vi "Refresh Limit Line.vi"(8 "error in (no error)":errorcluster, 10 "Item Names":string[][](array[string]), 11 "XY Graph":refnum<vi>) -> (0 "error out":errorcluster)   [LabVIEW 2020]
panel:
  out "XY Graph":cluster{dbl[], dbl[]}[](graph)
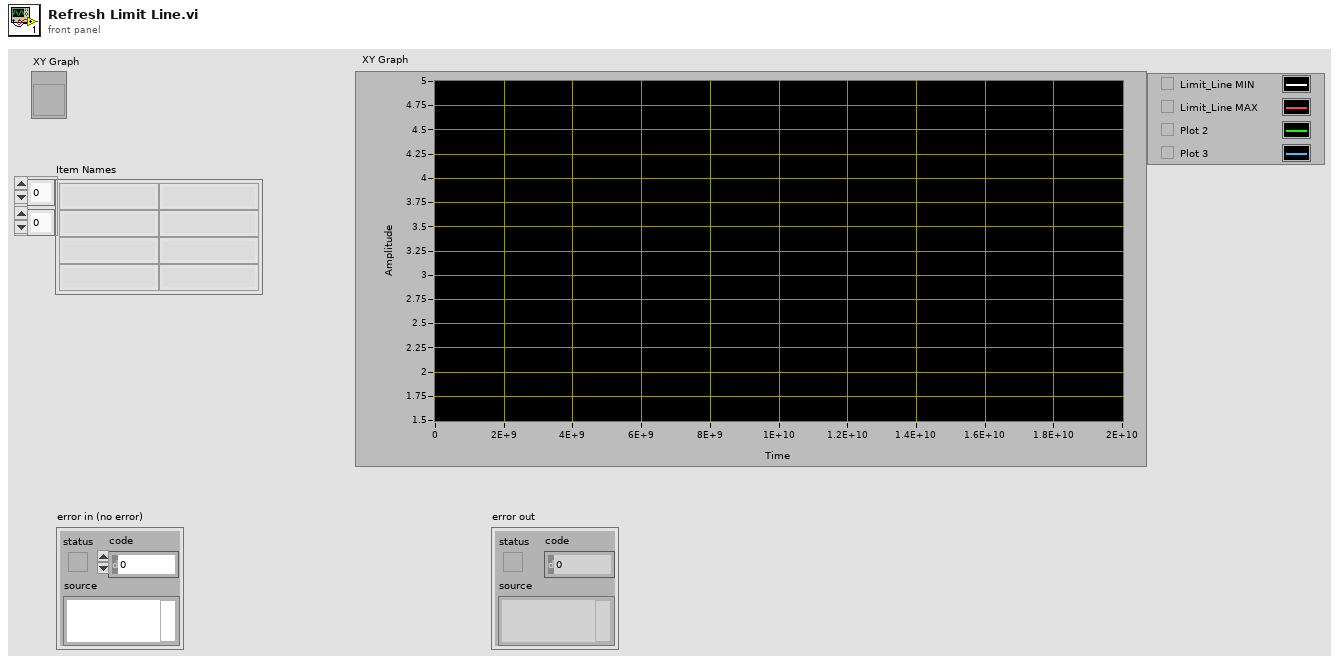
[diagram p1: front panel]
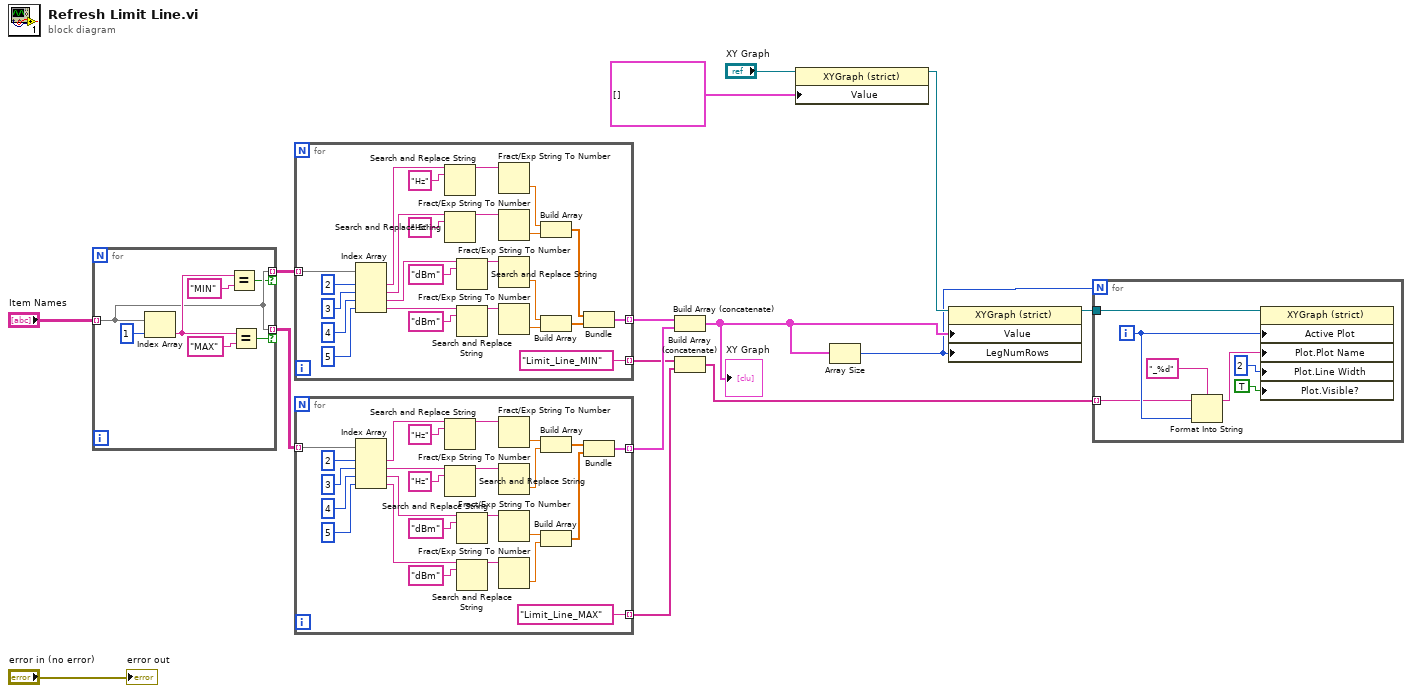
[diagram p0: block diagram]
diagram:
  n1 = for {
    tunnel: "Item Names" -> [w17] mode=indexing
    tunnel: [w17] -> w14 mode=indexing if=w20
    tunnel: [w17] -> w15 mode=indexing if=w16
    n2 = Index Array(array=w17, index=1) -> (element=w19:string)
    n3 = Equal?(x=w19, y="MIN") -> (x = y?=w16:bool)
    n4 = Equal?(x=w19, y="MAX") -> (x = y?=w20:bool)
  }
  n5 = for {
    tunnel: w15 -> [w47] mode=indexing
    tunnel: [w24] -> w6 mode=indexing
    tunnel: ["Limit_Line_MIN" ("format string")] -> w3 mode=indexing
    n6 = Index Array(array=w47, index #1=2 ("index"), index #2=3 ("index"), index #3=4 ("index"), index #4=5 ("index")) -> (element #1=w44:string, element #2=w39:string, element #3=w29:string, element #4=w28:string)
    n7 = Search and Replace String(input string=w44, search string="Hz") -> (result string=w42:string)  [unwired: 6 in, 3 out]
    n8 = Search and Replace String(input string=w39, search string="Hz") -> (result string=w41:string)  [unwired: 6 in, 3 out]
    n9 = Search and Replace String(input string=w29, search string="dBm") -> (result string=w31:string)  [unwired: 6 in, 3 out]
    n10 = Search and Replace String(input string=w28, search string="dBm") -> (result string=w32:string)  [unwired: 6 in, 3 out]
    n11 = Fract/Exp String To Number(string=w42) -> (number=w38:dbl)  [unwired: 3 in, 1 out]
    n12 = Fract/Exp String To Number(string=w41) -> (number=w37:dbl)  [unwired: 3 in, 1 out]
    n13 = Fract/Exp String To Number(string=w31) -> (number=w27:dbl)  [unwired: 3 in, 1 out]
    n14 = Fract/Exp String To Number(string=w32) -> (number=w26:dbl)  [unwired: 3 in, 1 out]
    n15 = Build Array(w38, w37) -> (w36:dbl[])
    n16 = Build Array(w27, w26) -> (w25:dbl[])
    n17 = Bundle(w36, w25) -> (w24:cluster{dbl[], dbl[]})  [unwired: 1 in]
  }
  n18 = for {
    tunnel: w14 -> [w72] mode=indexing
    tunnel: [w49] -> w5 mode=indexing
    tunnel: ["Limit_Line_MAX" ("format string")] -> w2 mode=indexing
    n19 = Index Array(array=w72, index #1=2 ("index"), index #2=3 ("index"), index #3=4 ("index"), index #4=5 ("index")) -> (element #1=w69:string, element #2=w64:string, element #3=w54:string, element #4=w53:string)
    n20 = Search and Replace String(input string=w69, search string="Hz") -> (result string=w67:string)  [unwired: 6 in, 3 out]
    n21 = Search and Replace String(input string=w64, search string="Hz") -> (result string=w66:string)  [unwired: 6 in, 3 out]
    n22 = Search and Replace String(input string=w54, search string="dBm") -> (result string=w56:string)  [unwired: 6 in, 3 out]
    n23 = Search and Replace String(input string=w53, search string="dBm") -> (result string=w57:string)  [unwired: 6 in, 3 out]
    n24 = Fract/Exp String To Number(string=w67) -> (number=w63:dbl)  [unwired: 3 in, 1 out]
    n25 = Fract/Exp String To Number(string=w66) -> (number=w62:dbl)  [unwired: 3 in, 1 out]
    n26 = Fract/Exp String To Number(string=w56) -> (number=w52:dbl)  [unwired: 3 in, 1 out]
    n27 = Fract/Exp String To Number(string=w57) -> (number=w51:dbl)  [unwired: 3 in, 1 out]
    n28 = Build Array(w63, w62) -> (w61:dbl[])
    n29 = Build Array(w52, w51) -> (w50:dbl[])
    n30 = Bundle(w61, w50) -> (w49:cluster{dbl[], dbl[]})  [unwired: 1 in]
  }
  n31 = Build Array (concatenate)(w6, w5) -> (w13:cluster{dbl[], dbl[]}[])
  "XY Graph" <- w13
  n32 = Build Array (concatenate)(w3, w2) -> (w1:string[])
  n33 = property class="XYGraph (strict)"(reference="XY Graph", "Value"=cluster{dbl[], dbl[]}[] []) -> (reference out=w8:refnum<vi>)  [unwired: 1 in, 1 out]
  n34 = Array Size(array=w13) -> (size(s)=w7:i32)
  n35 = property class="XYGraph (strict)"(reference=w8, "Value"=w13, "LegNumRows"=w7) -> (reference out=w4:refnum<vi>)  [unwired: 1 in, 1 out]
  n36 = for {
    N: w7 -> [_]
    tunnel: w4 -> [w79]
    tunnel: w1 -> [w73] mode=indexing
    i -> [w76]
    n37 = Format Into String(format string="_%d", initial string=w73, w76) -> (resulting string=w75:string)  [unwired: 1 in, 1 out]
    n38 = property class="XYGraph (strict)"(reference=w79, "Active Plot"=w76, "Plot.Plot Name"=w75, "Plot.Line Width"=u8 2, "Plot.Visible?"=TRUE ("Plot.Visible")) -> ()  [unwired: 1 in, 2 out]
  }
  "error out" <- "error in (no error)"
